vi "parse_gps_string.vi"(0 "data in":string) -> (1 "Time Stamp":timestamp, 2 "Latitude":dbl format="%#_20f", 3 "Longitude":dbl format="%#_20f")   [LabVIEW 2023]
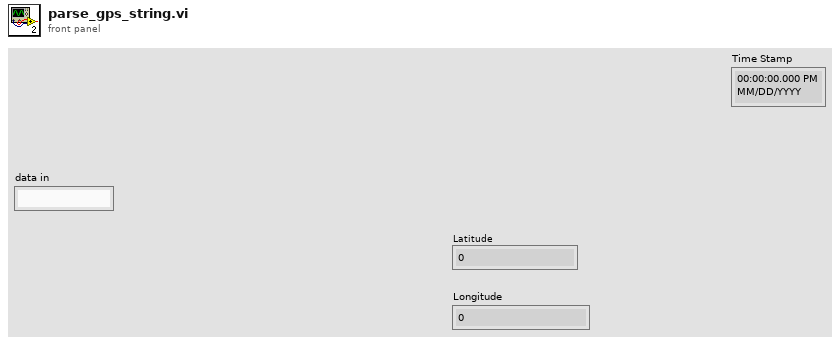
[diagram p1: front panel]
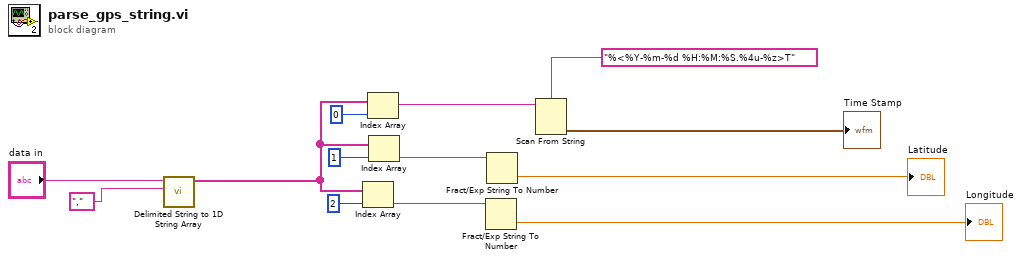
[diagram p0: block diagram]
diagram:
  n1 = call <vilib>:"Delimited String to 1D String Array.vi"("delimiter"=",", "delimited string"="data in") -> ("string array"=w11:string[])  [unwired: 9 in]
  n2 = Index Array(array=w11, index=2) -> (element=w13:string)
  n3 = Index Array(array=w11, index=0) -> (element=w5:string)
  n4 = Index Array(array=w11, index=1) -> (element=w12:string)
  n5 = Fract/Exp String To Number(string=w13) -> (number=→"Longitude":dbl)  [unwired: 3 in, 1 out]
  n6 = Fract/Exp String To Number(string=w12) -> (number=→"Latitude":dbl)  [unwired: 3 in, 1 out]
  n7 = Scan From String(format string="%<%Y-%m-%d %H:%M:%S.%4u-%z>T", input string=w5) -> (output 1=→"Time Stamp":timestamp)  [unwired: 3 in, 3 out]
